vi "ack.vi"(10 "n":dbl, 11 "m":dbl) -> (3 "Numeric":dbl)   [LabVIEW 2013]
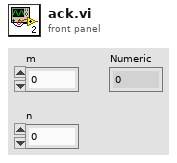
[diagram p1: front panel]
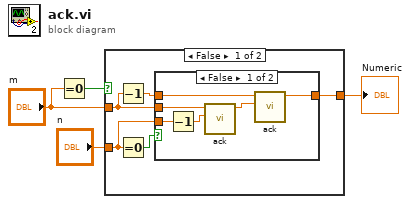
[diagram p0: block diagram]
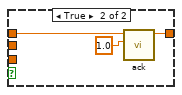
[diagram p2: hidden frame]
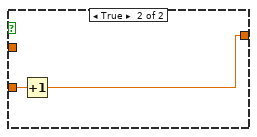
[diagram p3: hidden frame]
diagram:
  n1 = Equal To 0?(x="m") -> (x = 0?=w2:bool)
  n2 = case shown="False" w2 {
    tunnel: "n" -> [w7 w20]
    tunnel: [w8 w19] -> w3
    tunnel: "m" -> [w5 _]
    frame False {
      n3 = Decrement(x=w5) -> (x-1=w6:dbl)
      n4 = Equal To 0?(x=w7) -> (x = 0?=w9:bool)
      n5 = case shown="False" w9 {
        tunnel: [w10 w17] -> w8
        tunnel: w7 -> [w15 _]
        tunnel: w6 -> [w12 w16]
        tunnel: w5 -> [w11 _]
        frame False {
          n6 = Decrement(x=w15) -> (x-1=w14:dbl)
          n7 = call "ack.vi"("n"=w14, "m"=w11) -> ("Numeric"=w13:dbl)  [unwired: 9 in]
          n8 = call "ack.vi"("n"=w13, "m"=w12) -> ("Numeric"=w10:dbl)  [unwired: 9 in]
        }
        frame True {
          n9 = call "ack.vi"("n"=1.0, "m"=w16) -> ("Numeric"=w17:dbl)  [unwired: 9 in]
        }
      }
    }
    frame True {
      n10 = Increment(x=w20) -> (x+1=w19:dbl)
    }
  }
  "Numeric" <- w3
